vi "GetFrameStatistics.vi"(8 "error in (no error)":errorcluster) -> (0 "error out":errorcluster, 1 "FrameIn":u8[](array[numeric]), 2 "FrameNak":u8[](array[numeric]), 3 "FrameOut":u8[](array[numeric]))   [LabVIEW 2014]
uses:
  USBAnalyzerEllisysDll/Debug/USBAnalyzerEllisysDll.dll
panel:
  out "sizeFrameNak":i32
  out "sizeFrameOut":i32
  out "sizeFrameIn":i32
  out "return type":i32
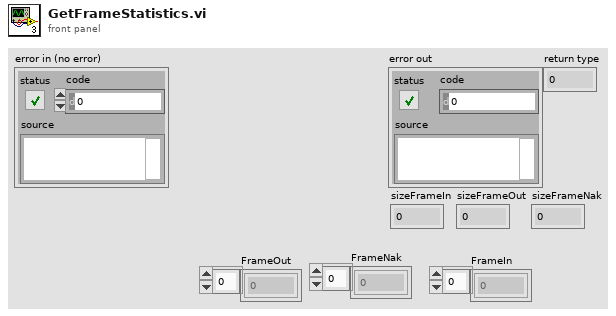
[diagram p1: front panel]
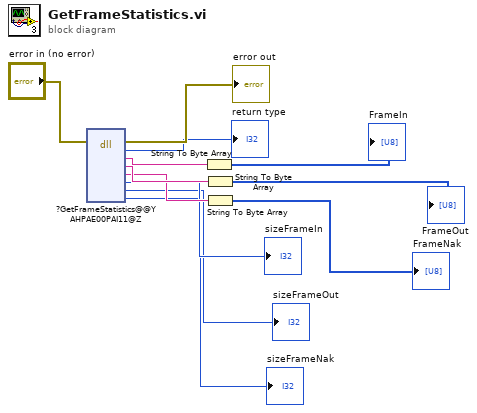
[diagram p0: block diagram]
diagram:
  n1 = dll-call lib="PTH2labs CUsersMichał\tDocumentsEllisysAnalyzerUSBAnalyzerEllisysDllDebugUSBAnalyzerEllisysDll.dll" fn="?GetFrameStatistics@@YAHPAE00PAI11@Z"(error in="error in (no error)") -> (error out=→"error out":errorcluster, "return type"=→"return type":i32, "frameIn"=w9:string, "frameOut"=w8:string, "frameNak"=w7:string, "sizeFrameIn"=→"sizeFrameIn":i32, "sizeFrameOut"=→"sizeFrameOut":i32, "sizeFrameNak"=→"sizeFrameNak":i32)  [unwired: 8 in, 1 out]
  n2 = String To Byte Array(string=w9) -> (unsigned byte array=→"FrameIn":u8[])
  n3 = String To Byte Array(string=w8) -> (unsigned byte array=→"FrameOut":u8[])
  n4 = String To Byte Array(string=w7) -> (unsigned byte array=→"FrameNak":u8[])
